vi "Equal To Core Actor.vi"(7 "Actor":refnum<class "Actor.lvclass">) -> (2 "Core Actor":bool)   [LabVIEW 2025, in "jettl.lvlib" / "Actor.lvlib"]
uses:
  Actor.lvlib
  Actor/Actor.lvclass
  Core Actor/Core Actor.lvclass
  C:/git/jettl/src/jettl/jettl/Actor/Actor/Actor.lvclass
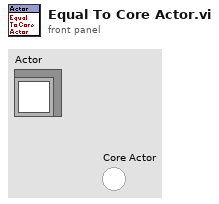
[diagram p1: front panel]
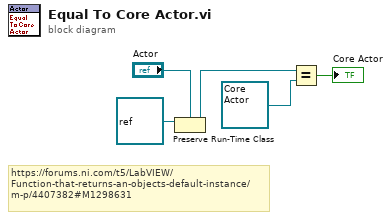
[diagram p0: block diagram]
diagram:
  # "https://forums.ni.com/t5/LabVIEW/Function-that-returns-an-objects-default-instance/m-p/4407382#M1298631"
  n1 = Preserve Run-Time Class(object in=refnum<class> refnum ("LabVIEW Object"), 2:"Actor") -> (object out=w3:refnum<class "Actor.lvclass">)  [unwired: 1 in, 1 out]
  n2 = Equal?(x=w3, y=refnum<class "Core Actor.lvclass"> refnum ("jettl.lvlib:Actor.lvlib:Core Actor.lvclass")) -> (x = y?=→"Core Actor":bool)
